vi "seven segment try.vi"() -> ()   [LabVIEW 2020]
panel:
  out "1":bool
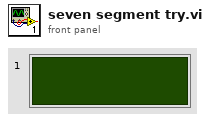
[diagram p1: front panel]
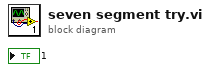
[diagram p0: block diagram]
diagram:
